vi "Change Project Prefix.vi"() -> ()   [LabVIEW 2015]
panel:
  in  "Template Path":path
  in  "New Prefix":string="Shit"
  in  "Old Prefix":string="LocTask"
  out "Dependency Paths":path[](array[path])
  # "1. Duplicate project, selecting only the dependencies in the LV Source folder hierarchy\n2. Open new project, make sure LV Source is included as populating folder\n3. Edit the icon template\n4. Select the main VI\n5. Run this VI"
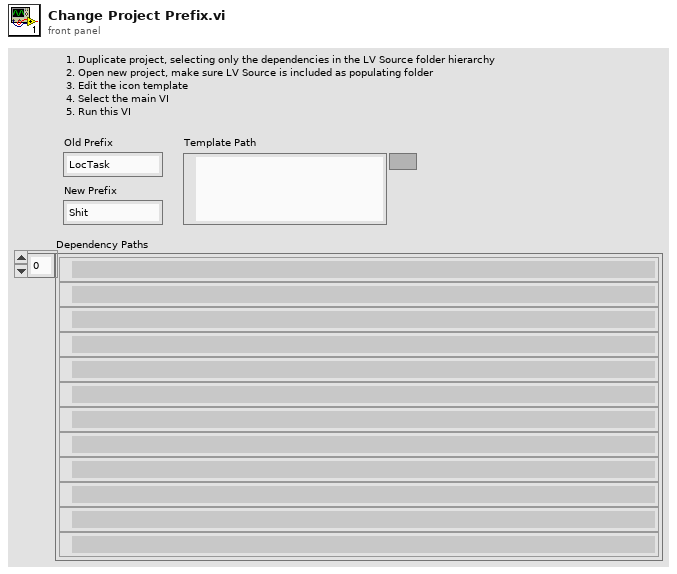
[diagram p1: front panel]
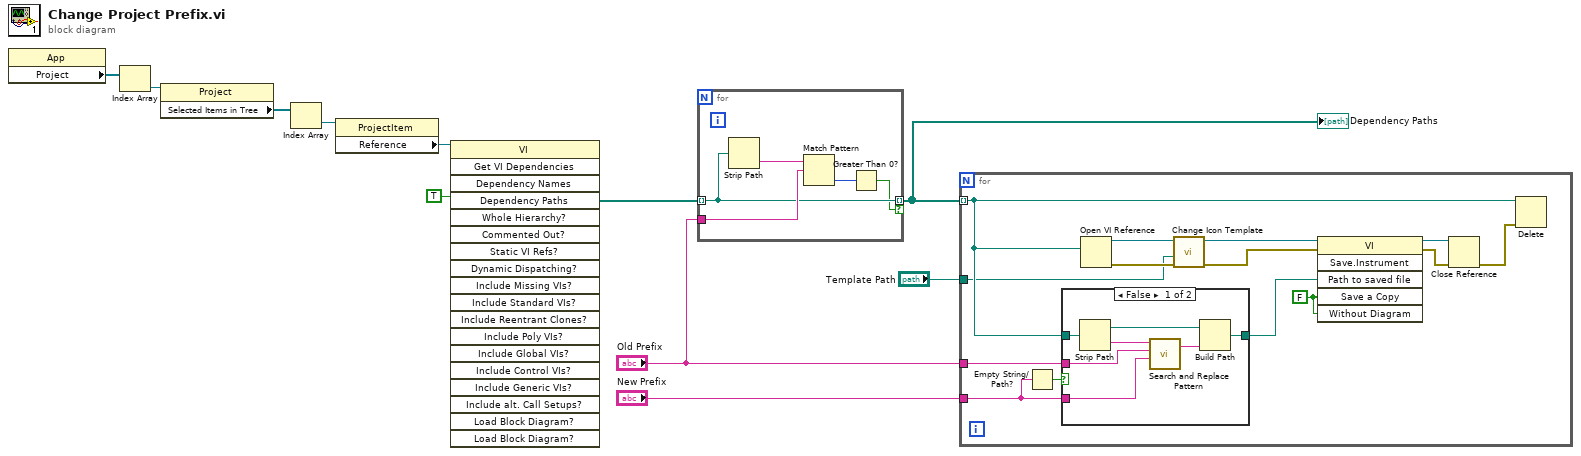
[diagram p0: block diagram]
diagram:
  n1 = property class="App"() -> ("Project"=w7:refnum<vi>[])  [unwired: 2 in, 2 out]
  n2 = Index Array(array=w7) -> (element=w6:refnum<vi>)  [unwired: 1 in]
  n3 = property class="Project"(reference=w6) -> ("Selected Items in Tree"=w5:refnum<vi>[])  [unwired: 1 in, 2 out]
  n4 = Index Array(array=w5) -> (element=w4:refnum<vi>)  [unwired: 1 in]
  n5 = property class="ProjectItem"(reference=w4) -> ("Reference"=w3:refnum<vi>)  [unwired: 1 in, 2 out]
  n6 = invoke class="VI" method="Get VI Dependencies"(reference=w3, "Whole Hierarchy?"=TRUE) -> ("Dependency Paths"=w11:path[])  [unwired: 17 in, 18 out]
  n7 = for {
    tunnel: w11 -> [w14] mode=indexing
    tunnel: "Old Prefix" -> [w15]
    tunnel: [w14] -> w10 mode=indexing if=w12
    n8 = Strip Path(path=w14) -> (name=w16:string)  [unwired: 1 out]
    n9 = Match Pattern(string=w16, regular expression=w15) -> (offset past match=w13:i32)  [unwired: 1 in, 3 out]
    n10 = Greater Than 0?(x=w13) -> (x > 0?=w12:bool)
  }
  "Dependency Paths" <- w10
  n11 = for {
    tunnel: w10 -> [w25] mode=indexing
    tunnel: "Old Prefix" -> [w30]
    tunnel: "New Prefix" -> [w19]
    tunnel: "Template Path" -> [w20]
    w17 = FALSE ("Save a Copy")
    n12 = Empty String/Path?(string/path=w19) -> (empty?=w18:bool)
    n13 = case shown="False" w18 {
      tunnel: w30 -> [w36 _]
      tunnel: w19 -> [w35 _]
      tunnel: [w32 w38] -> w29
      tunnel: w25 -> [w31 w38]
      frame False {
        n14 = Strip Path(path=w31) -> (stripped path=w34:path, name=w37:string)
        n15 = call <vilib>:"Search and Replace Pattern.vi"("string"=w37, "regular expression (\"\")"=w36, "replace string (\"\")"=w35) -> ("result string"=w33:string)  [unwired: 2 in, 1 out]
        n16 = Build Path(base path=w34, name or relative path=w33) -> (appended path=w32:path)
      }
      frame True {
      }
    }
    n17 = Open VI Reference(vi path=w25) -> (vi reference=w24:refnum<vi>, error out=w23:errorcluster)  [unwired: 5 in]
    n18 = call "Change Icon Template.vi"("error in (no error)"=w23, "Template Path"=w20, "vi reference"=w24) -> ("error out"=w21:errorcluster, "reference out"=w22:refnum<vi>)  [unwired: 7 in]
    n19 = invoke class="VI" method="Save.Instrument"(reference=w22, error in=w21, "Path to saved file"=w29, "Save a Copy"=w17, "Without Diagram"=w17) -> (reference out=w28:refnum<vi>, error out=w27:errorcluster)  [unwired: 1 in, 4 out]
    n20 = Close Reference(reference=w28, error in (no error)=w27) -> (error out=w26:errorcluster)
    n21 = Delete(path (use dialog)=w25, error in=w26) -> ()  [unwired: 3 in, 3 out]
  }
